vi "Process.Report.vi"(8 "Error":errorcluster, 10 "Stop on Error?":bool, 11 "Process in":refnum<class "Process.lvclass">) -> (2 "Stop":bool, 3 "Process out":refnum<class "Process.lvclass">)   [LabVIEW 2015, in "VS Inline Async API.lvlib" / "Process.lvclass"]
uses:
  Process.lvclass
  Process.lvclass/Process.ctl
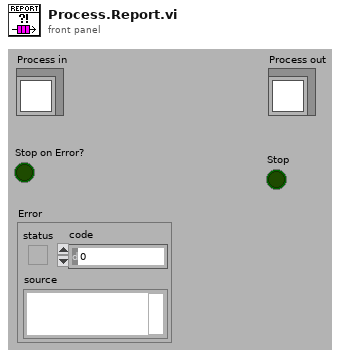
[diagram p1: front panel]
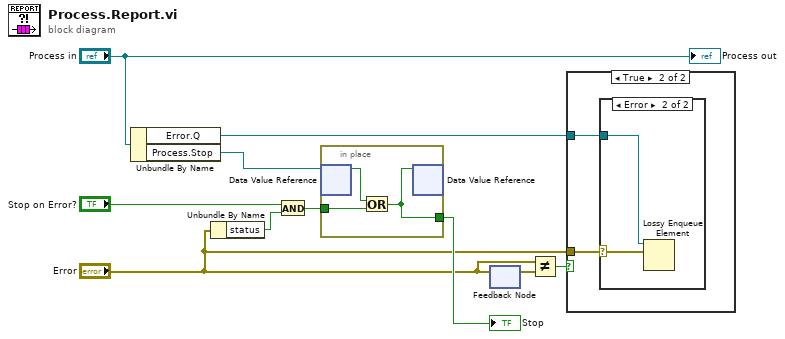
[diagram p0: block diagram]
diagram:
  n1 = Unbundle By Name("Process in") -> ("Error.Q"=w7:refnum<queue>, "Process.Stop"=w1:refnum<data-value>)
  n2 = Unbundle By Name("Error") -> ("status"=w5:bool)
  n3 = And(x="Stop on Error?", y=w5) -> (x .and. y?=w4:bool)
  n4 = in-place {
    in-place-border: [w11] -> w3
    in-place-border: w4 -> [w12]
    n5 = in-place-dvr #1(w1) -> (w13:bool)  [unwired: 1 out]
    n6 = Or(x=w13, y=w12) -> (x .or. y?=w11:bool)
    n7 = in-place-dvr #1(w11) -> ()  [unwired: 2 out]
  }
  "Stop" <- w3
  n8 = feedback #2() -> (w9:errorcluster)  [unwired: 1 in]
  n9 = feedback-in #2("Error") -> ()
  n10 = Not Equal?(x="Error", y=w9) -> (x != y?=w10:bool)
  n11 = case shown="True" w10 {
    tunnel: w7 -> [_ w15]
    tunnel: "Error" -> [_ w14]
    frame False {
    }
    frame True {
      n12 = case shown="Error" w14 {
        selector: w14 -> [_ w16]
        tunnel: w15 -> [_ w17]
        frame No Error {
        }
        frame Error {
          n13 = Lossy Enqueue Element(queue=w17, element=w16) -> ()  [unwired: 1 in, 4 out]
        }
      }
    }
  }
  "Process out" <- "Process in"
